vi "LC Global.vi"(7 "Mode":T3, 8 "error in (no error)":errorcluster caption="Error In", 9 "Write":T1) -> (0 "error out":errorcluster caption="Error Out", 2 "Read":T1[](array[typedef]), 3 "VI Info":T2)   [LabVIEW 2020]
uses:
  LC Mode.ctl
  LC Single Control Information.ctl
  LC Control Information.ctl
  <vilib>/Utility/xml.llb/Read From XML File(string).vi
  <vilib>/Utility/xml.llb/Write to XML File(string).vi
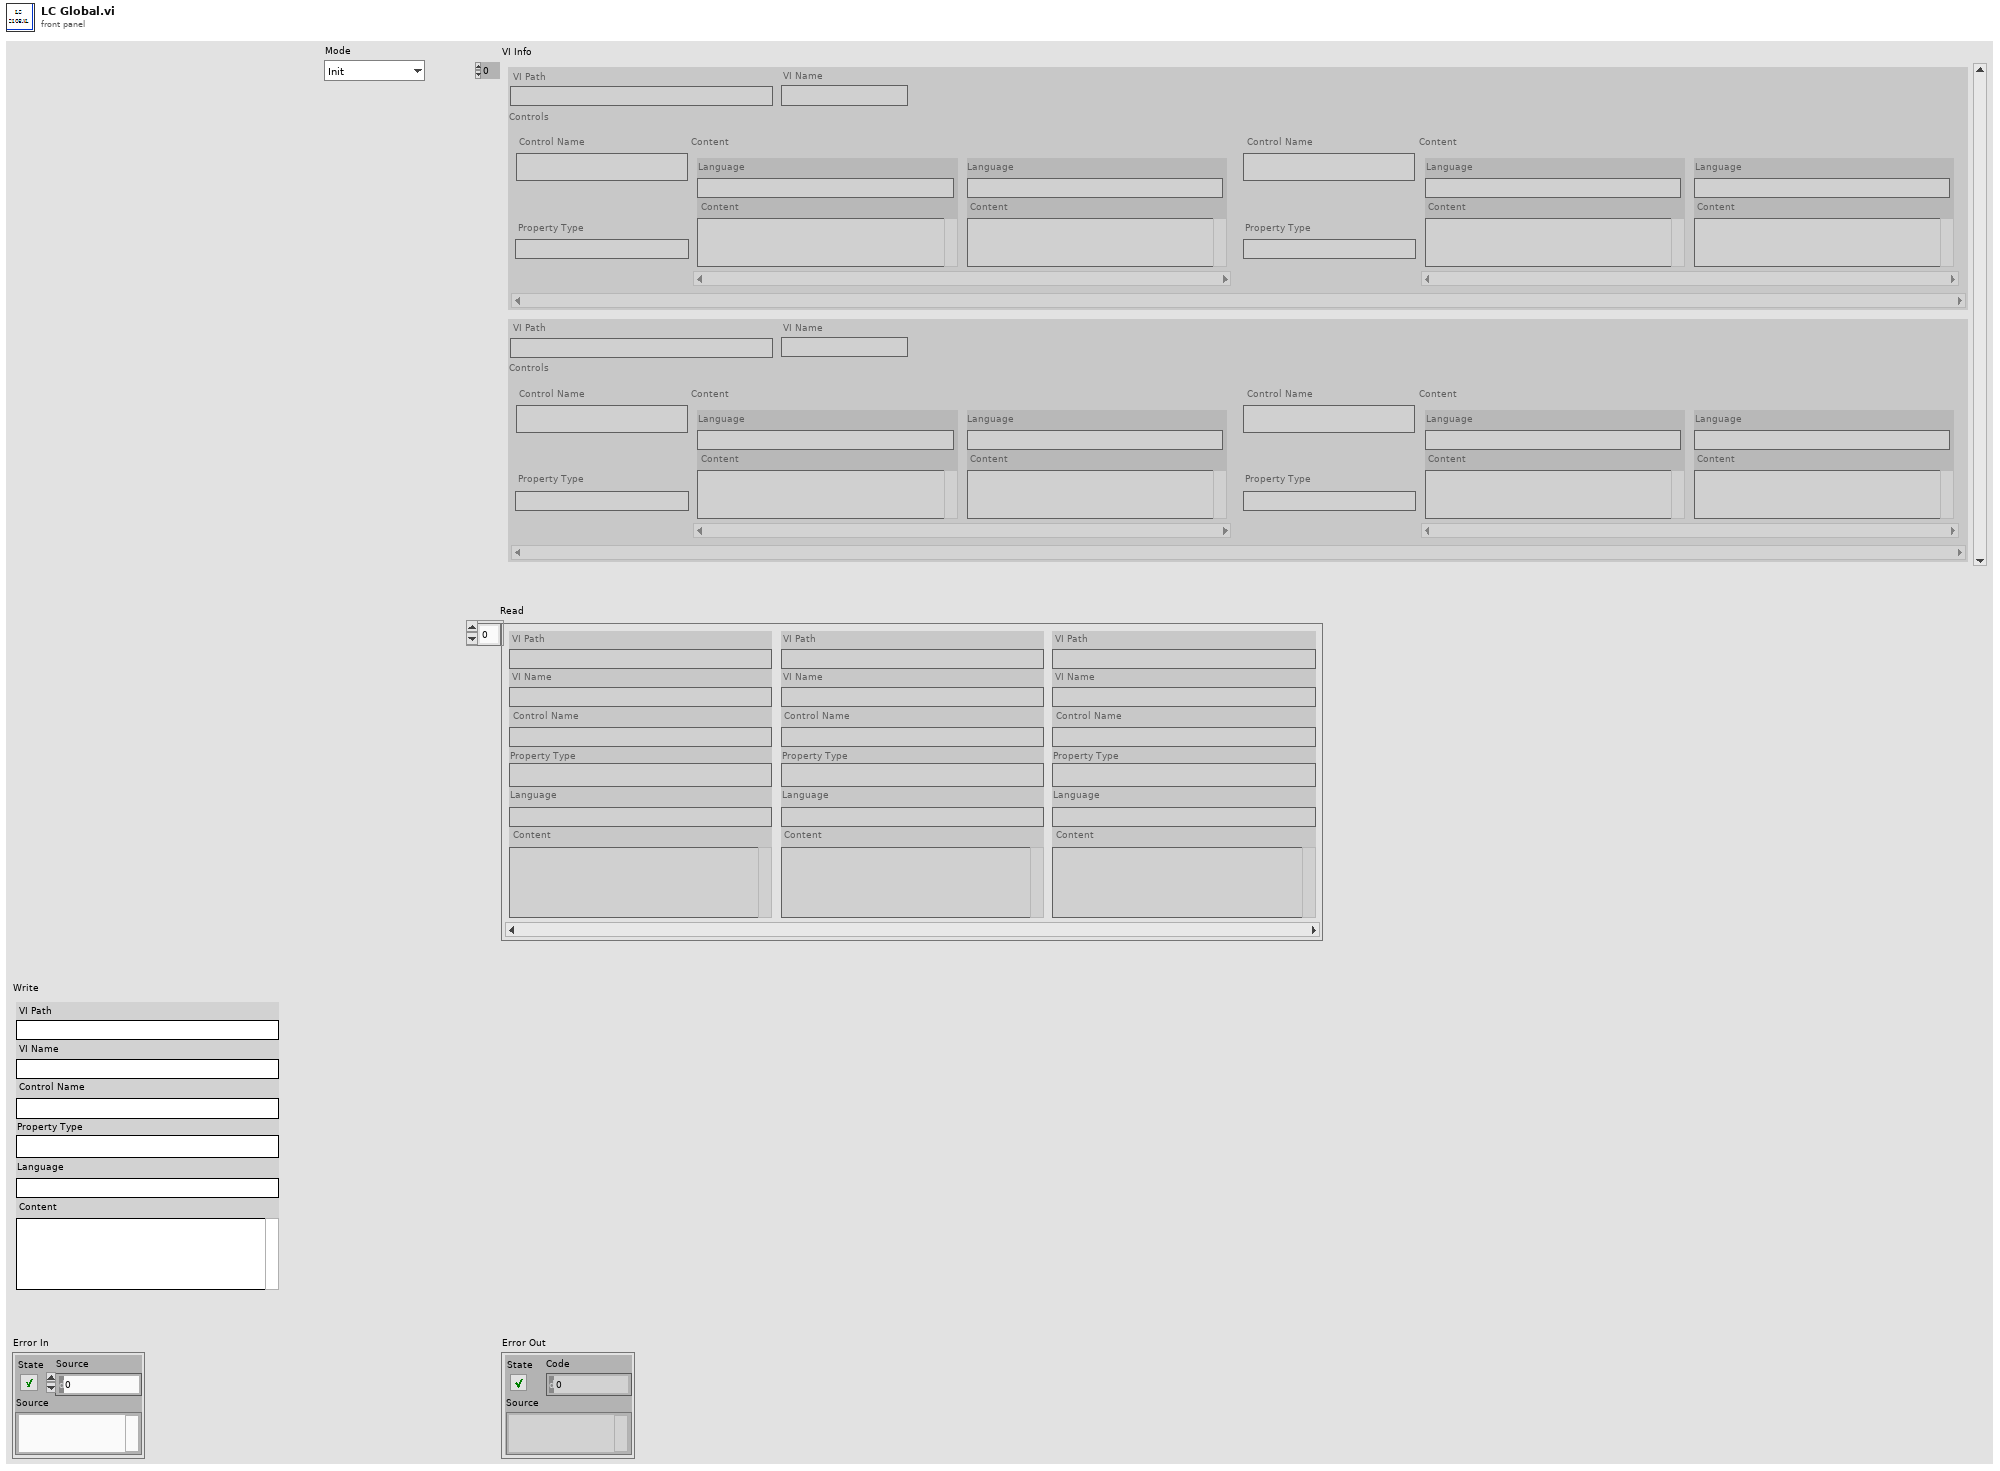
[diagram p1: front panel]
types:
  T1 = typedef "LC Single Control Information.ctl" = cluster{"VI Path":string, "VI Name":string, "Control Name":string, "Property Type":string, "Language":string, "Content":string}
  T2 = typedef "LC Control Information.ctl" = cluster{"Controls":cluster{"Control Name":string, "Property Type":string, "Content":cluster{"Language":string, "Content":string}[]}[], "VI Path":string, "VI Name":string}[]
  T3 = typedef "LC Mode.ctl" = enum16{"Init", "NONE", "Read", "Write", "Delete", "Clear", "Save"}
  T4 = cluster{"Control Name":string, "Property Type":string, "Content":cluster{"Language":string, "Content":string}[]}[]
  T5 = cluster{"Controls":cluster{"Control Name":string, "Property Type":string, "Content":cluster{"Language":string, "Content":string}[]}[], "VI Path":string, "VI Name":string}
  T6 = cluster{"Control Name":string, "Property Type":string, "Content":cluster{"Language":string, "Content":string}[]}
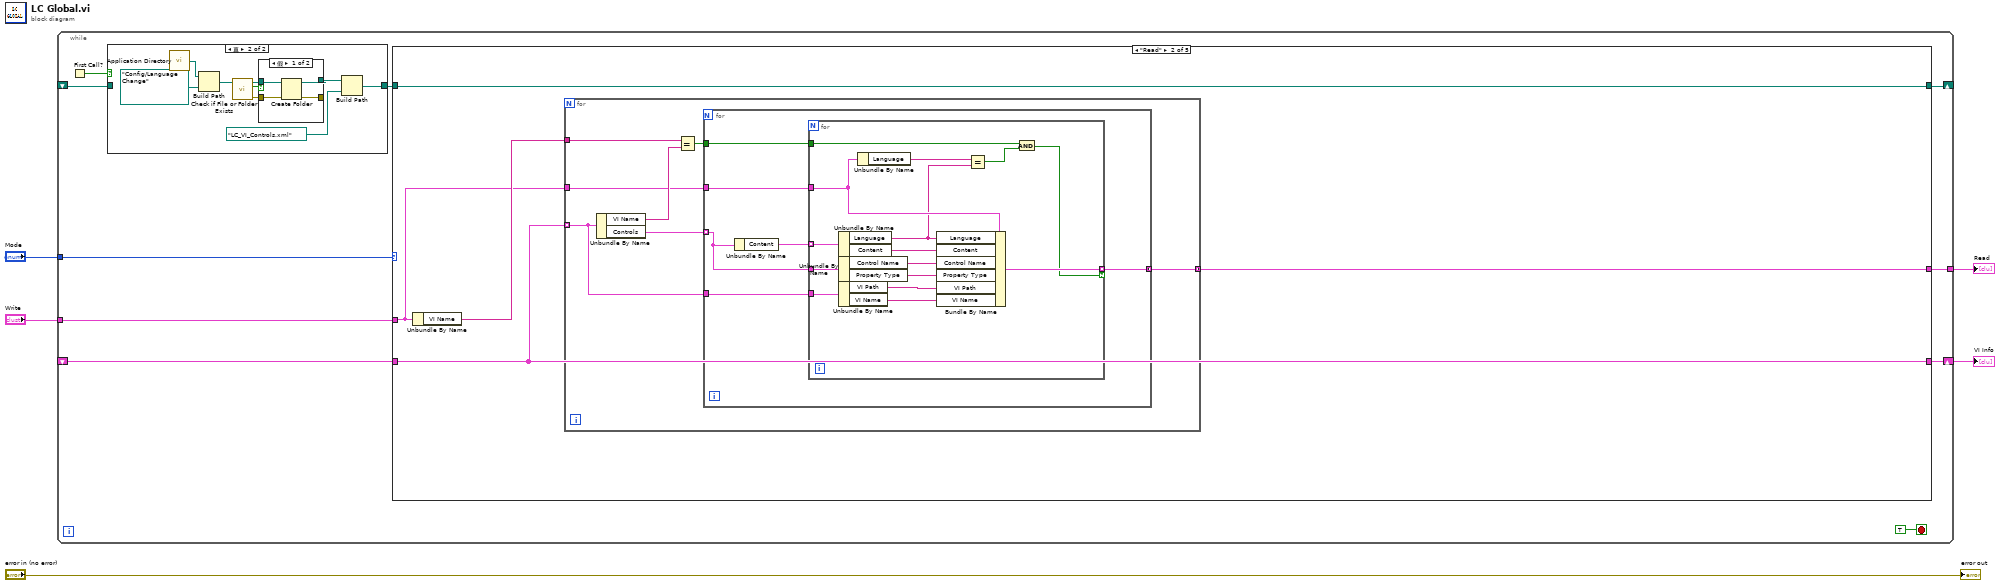
[diagram p0: block diagram]
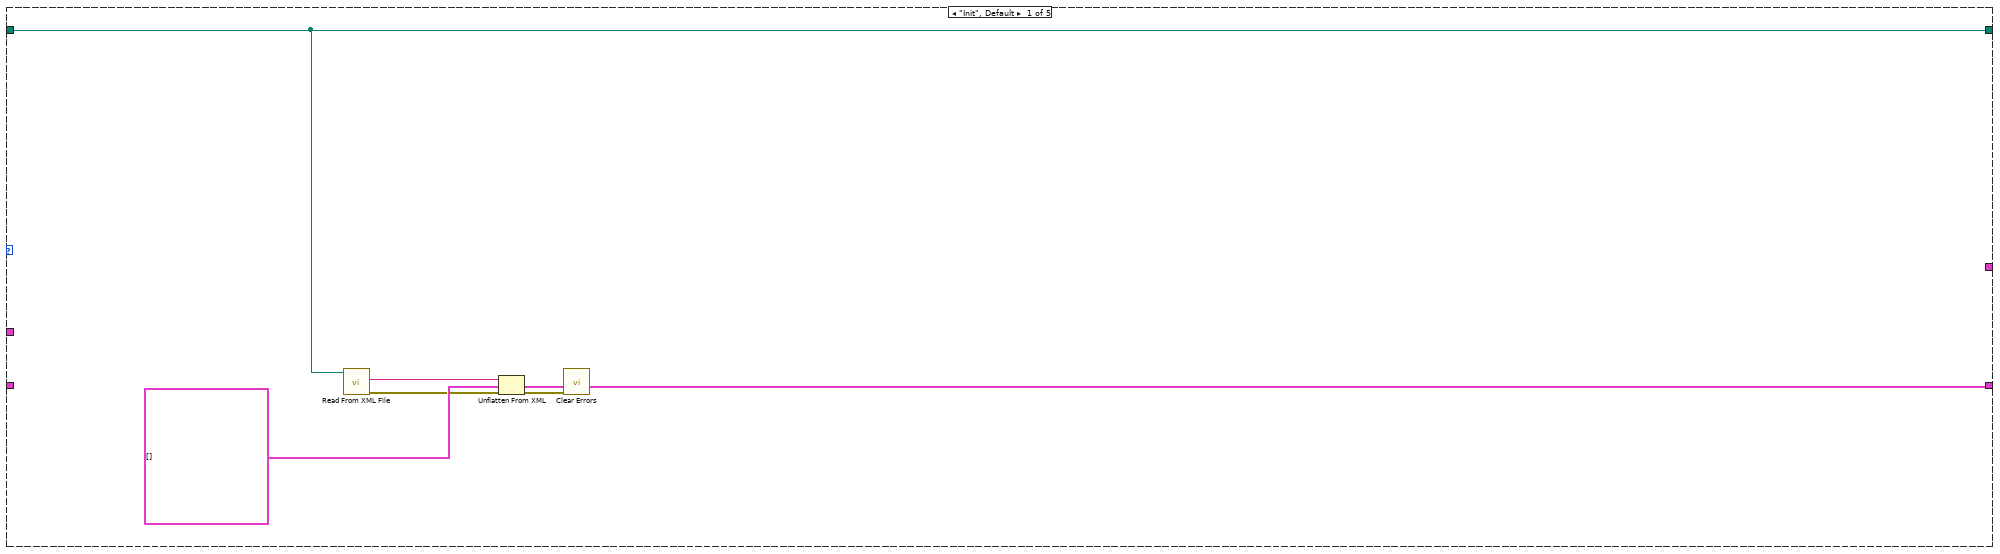
[diagram p4: hidden frame]
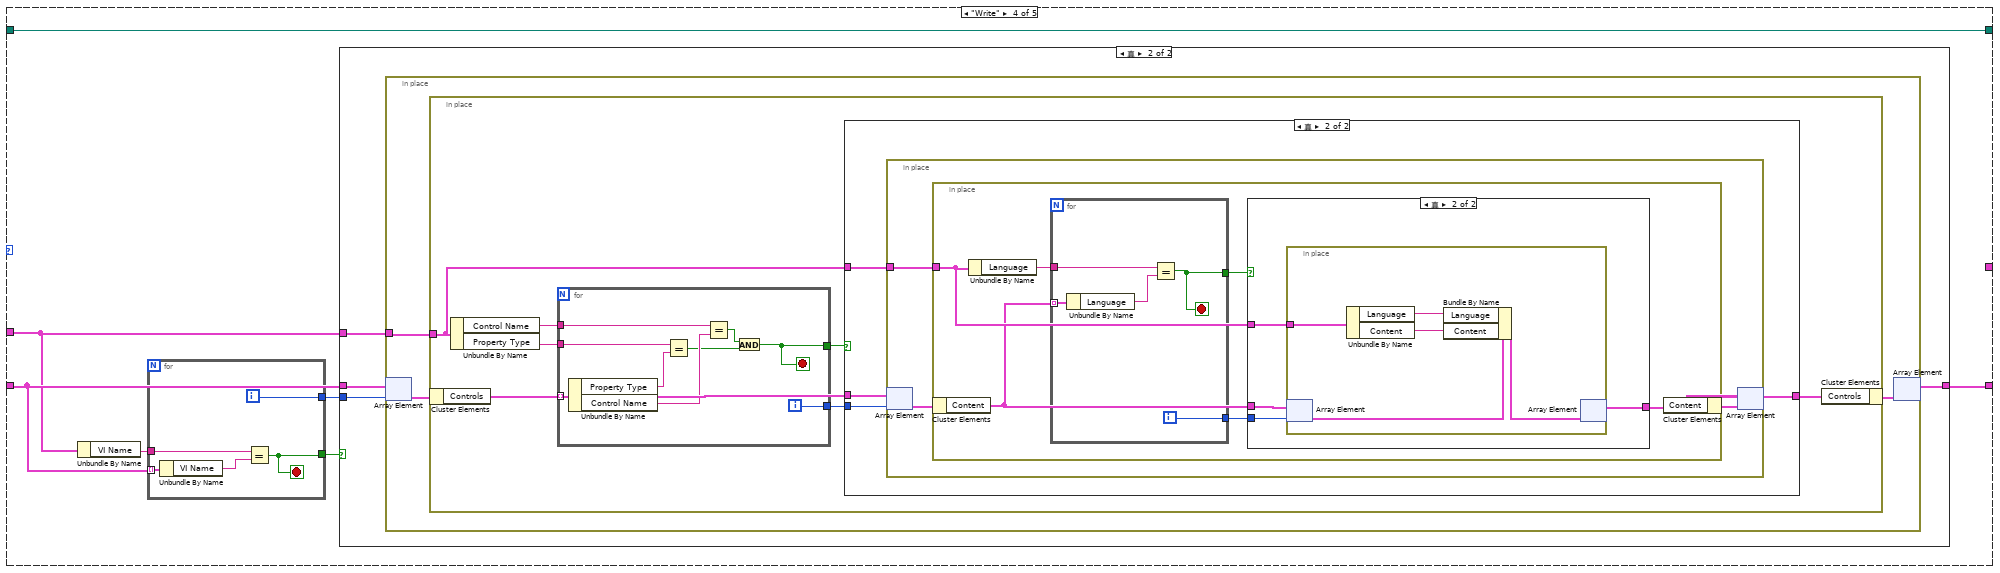
[diagram p6: hidden frame]
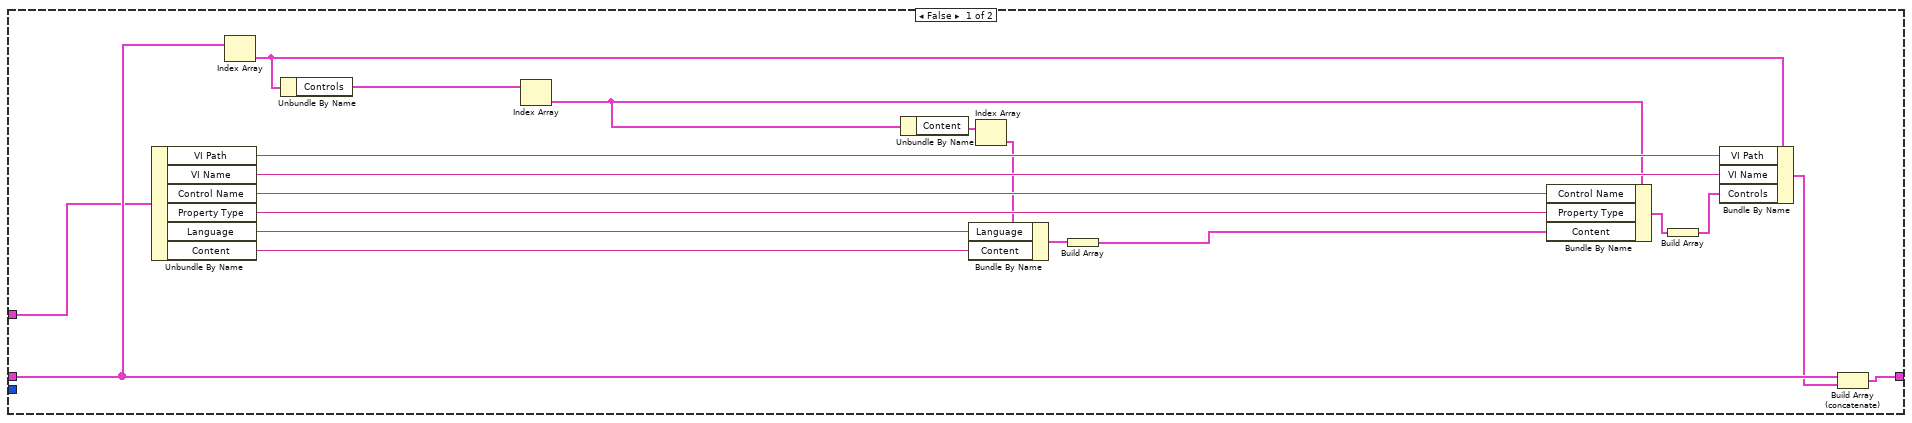
[diagram p7: hidden frame]
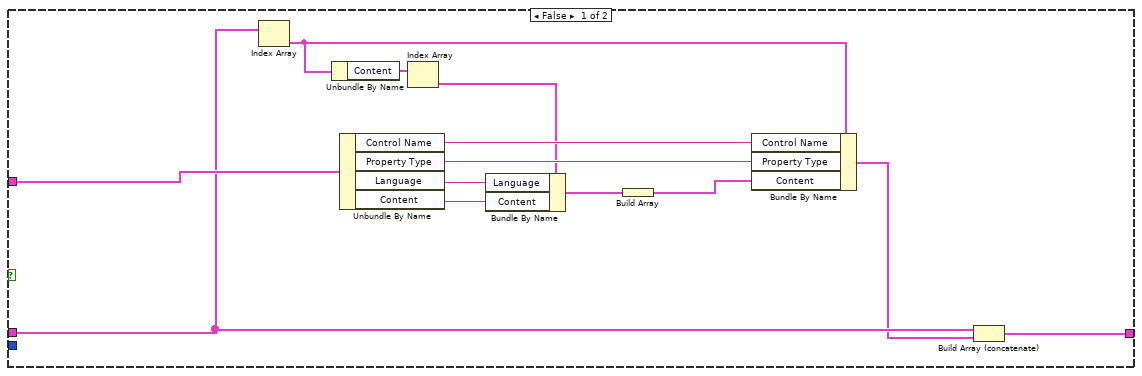
[diagram p8: hidden frame]
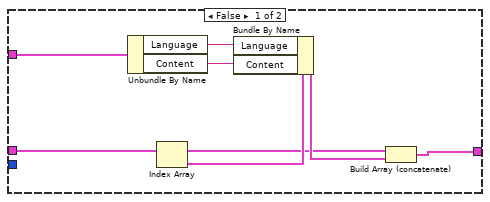
[diagram p9: hidden frame]
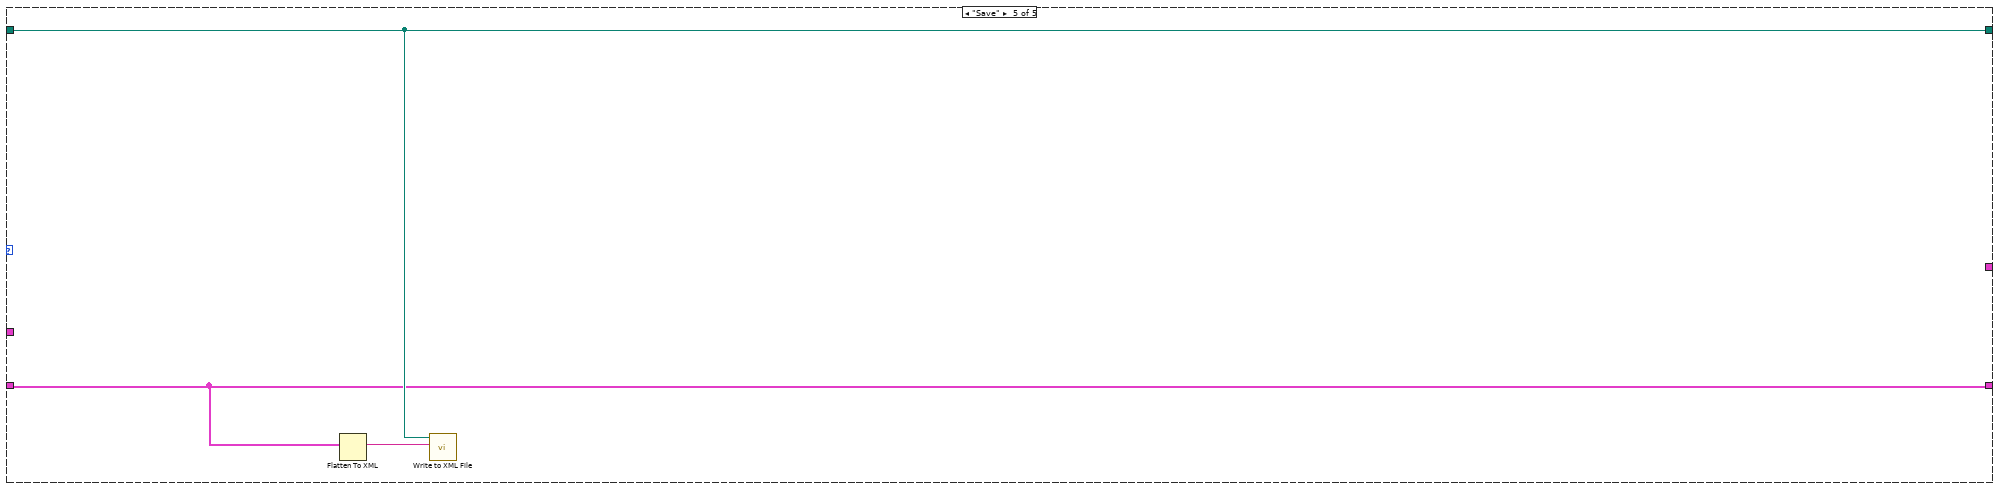
[diagram p10: hidden frame]
diagram:
  n1 = while {
    tunnel: "Mode" -> [w15]
    shift-right: [w13] -> _
    shift-left: _ -> [w8]
    shift-right: [w12] -> w2
    shift-left: _ -> [w11]
    tunnel: "Write" -> [w7]
    tunnel: [w6] -> w1
    stop <- TRUE stop-if-true
    n2 = First Call?() -> (First Call?: T/F=w10:bool)
    n3 = case shown="真" w10 {
      tunnel: [w16 w17] -> w9
      tunnel: w8 -> [w16 _]
      frame False {
      }
      frame True {
        n4 = call <vilib>:"Application Directory.vi"() -> ("Application Directory"=w25:path)
        n5 = Build Path(base path=w25, name or relative path=path "Config/Language Change" ("名称或相对路径")) -> (appended path=w23:path)
        n6 = call <vilib>:"Check if File or Folder Exists.vi"("path"=w23) -> ("error out"=w20:errorcluster, "file or folder exists?"=w22:bool, "dup path"=w21:path)  [unwired: 8 in]
        n7 = case shown="假" w22 {
          tunnel: w21 -> [w29 w31]
          tunnel: w20 -> [w28 w30]
          tunnel: [w27 w31] -> w19
          tunnel: [w26 w30] -> _
          frame False {
            n8 = Create Folder(path (use dialog)=w29, error in=w28) -> (created path=w27:path, error out=w26:errorcluster)  [unwired: 1 in, 1 out]
          }
          frame True {
          }
        }
        n9 = Build Path(base path=w19, name or relative path=path "LC_VI_Controls.xml" ("名称或相对路径")) -> (appended path=w17:path)
      }
    }
    n10 = case shown="\"Read\"" w15 {
      tunnel: [w37 w42 w72 w79 w175] -> w13
      tunnel: w9 -> [w37 w42 w72 w79 w175]
      tunnel: [w35 w40 w71 w73 w174] -> w12
      tunnel: w11 -> [_ w40 w71 w76 w174]
      tunnel: w7 -> [_ w39 _ w74 _]
      tunnel: [_ w38 _ _ _] -> w6
      frame "Init", Default {
        n11 = call-poly <vilib>:"Read From XML File.vi"("XML File Path"=w37) -> ("error out"=w33:errorcluster, "XML Elements"=w36:string)  [unwired: 8 in, 1 out]
        n12 = Unflatten From XML(xml string=w36, type=T2 [] ("VI Info"), error in (no error)=w33) -> (value=w35:T2, error out=w32:errorcluster)
        n13 = call <vilib>:"Clear Errors.vi"("error in (no error)"=w32) -> ()  [unwired: 5 in, 2 out]
      }
      frame "Read" {
        n14 = Unbundle By Name(w39) -> ("VI Name"=w41:string)
        n15 = for {
          tunnel: w41 -> [w48]
          tunnel: w40 -> [w44] mode=indexing
          tunnel: w39 -> [w45]
          tunnel: [w43] -> w38 mode=concatenating
          n16 = Unbundle By Name(w44) -> ("VI Name"=w49:string, "Controls"=w47:T4)
          n17 = Equal?(x=w48, y=w49) -> (x = y?=w46:bool)
          n18 = for {
            tunnel: w47 -> [w53] mode=indexing
            tunnel: w46 -> [w51]
            tunnel: w45 -> [w54]
            tunnel: w44 -> [w52]
            tunnel: [w50] -> w43 mode=concatenating
            n19 = Unbundle By Name(w53) -> ("Content"=w55:cluster{"Language":string, "Content":string}[])
            n20 = for {
              tunnel: w55 -> [w70] mode=indexing
              tunnel: w54 -> [w62]
              tunnel: w53 -> [w68]
              tunnel: w52 -> [w65]
              tunnel: w51 -> [w58]
              tunnel: [w57] -> w50 mode=indexing if=w56
              n21 = Unbundle By Name(w70) -> ("Language"=w60:string, "Content"=w69:string)
              n22 = Unbundle By Name(w68) -> ("Control Name"=w67:string, "Property Type"=w66:string)
              n23 = Unbundle By Name(w65) -> ("VI Path"=w64:string, "VI Name"=w63:string)
              n24 = Unbundle By Name(w62) -> ("Language"=w61:string)
              n25 = Bundle By Name(cluster=w62, "Language"=w60, "Content"=w69, "Control Name"=w67, "Property Type"=w66, "VI Path"=w64, "VI Name"=w63) -> (w57:T1)
              n26 = Equal?(x=w61, y=w60) -> (x = y?=w59:bool)
              n27 = And(x=w58, y=w59) -> (x .and. y?=w56:bool)
            }
          }
        }
      }
      frame "NONE" {
      }
      frame "Write" {
        n28 = Unbundle By Name(w74) -> ("VI Name"=w78:string)
        n29 = for {
          tunnel: w76 -> [w173] mode=indexing
          tunnel: w78 -> [w172]
          tunnel: [w170] -> w77
          tunnel: [w169] -> w75
          i -> [w169]
          stop <- w170 stop-if-true
          n30 = Unbundle By Name(w173) -> ("VI Name"=w171:string)
          n31 = Equal?(x=w172, y=w171) -> (x = y?=w170:bool)
        }
        n32 = case shown="真" w77 {
          tunnel: w76 -> [w98 w102]
          tunnel: w75 -> [_ w101]
          tunnel: w74 -> [w97 w100]
          tunnel: [w80 w99] -> w73
          frame False {
            n33 = Unbundle By Name(w97) -> ("VI Path"=w96:string, "VI Name"=w95:string, "Control Name"=w92:string, "Property Type"=w91:string, "Language"=w87:string, "Content"=w86:string)
            n34 = Index Array(array=w98) -> (element=w94:T5)  [unwired: 1 in]
            n35 = Unbundle By Name(w94) -> ("Controls"=w93:T4)
            n36 = Index Array(array=w93) -> (element=w90:T6)  [unwired: 1 in]
            n37 = Unbundle By Name(w90) -> ("Content"=w89:cluster{"Language":string, "Content":string}[])
            n38 = Index Array(array=w89) -> (element=w88:cluster{"Language":string, "Content":string})  [unwired: 1 in]
            n39 = Bundle By Name(cluster=w88, "Language"=w87, "Content"=w86) -> (w85:cluster{"Language":string, "Content":string})
            n40 = Build Array(w85) -> (w84:cluster{"Language":string, "Content":string}[])
            n41 = Bundle By Name(cluster=w90, "Control Name"=w92, "Property Type"=w91, "Content"=w84) -> (w83:T6)
            n42 = Build Array(w83) -> (w82:T4)
            n43 = Bundle By Name(cluster=w94, "VI Path"=w96, "VI Name"=w95, "Controls"=w82) -> (w81:T5)
            n44 = Build Array (concatenate)(w98, w81) -> (w80:T2)
          }
          frame True {
            n45 = in-place {
              in-place-border: w100 -> [w105]
              n46 = in-place-array #1(w102, w101) -> (w104:T5)
              n47 = in-place {
                in-place-border: w105 -> [w109]
                n48 = in-place-cluster #2(w104) -> ("Controls"=w107:T4)
                n49 = Unbundle By Name(w109) -> ("Control Name"=w112:string, "Property Type"=w108:string)
                n50 = for {
                  tunnel: w107 -> [w168] mode=indexing
                  tunnel: w112 -> [w167]
                  tunnel: [w165] -> w110
                  tunnel: [w160] -> w111
                  tunnel: w108 -> [w164]
                  i -> [w165]
                  stop <- w160 stop-if-true
                  n51 = Unbundle By Name(w168) -> ("Property Type"=w163:string, "Control Name"=w166:string)
                  n52 = Equal?(x=w164, y=w163) -> (x = y?=w161:bool)
                  n53 = Equal?(x=w167, y=w166) -> (x = y?=w162:bool)
                  n54 = And(x=w162, y=w161) -> (x .and. y?=w160:bool)
                }
                n55 = case shown="真" w111 {
                  tunnel: w110 -> [_ w127]
                  tunnel: w107 -> [w115 w128]
                  tunnel: w109 -> [w125 w129]
                  tunnel: [w113 w126] -> w106
                  frame False {
                    n56 = Index Array(array=w115) -> (element=w122:T6)  [unwired: 1 in]
                    n57 = Unbundle By Name(w122) -> ("Content"=w121:cluster{"Language":string, "Content":string}[])
                    n58 = Unbundle By Name(w125) -> ("Control Name"=w124:string, "Property Type"=w123:string, "Language"=w119:string, "Content"=w118:string)
                    n59 = Index Array(array=w121) -> (element=w120:cluster{"Language":string, "Content":string})  [unwired: 1 in]
                    n60 = Bundle By Name(cluster=w120, "Language"=w119, "Content"=w118) -> (w117:cluster{"Language":string, "Content":string})
                    n61 = Build Array(w117) -> (w116:cluster{"Language":string, "Content":string}[])
                    n62 = Bundle By Name(cluster=w122, "Control Name"=w124, "Property Type"=w123, "Content"=w116) -> (w114:T6)
                    n63 = Build Array (concatenate)(w115, w114) -> (w113:T4)
                  }
                  frame True {
                    n64 = in-place {
                      in-place-border: w129 -> [w132]
                      n65 = in-place-array #3(w128, w127) -> (w131:T6)
                      n66 = in-place {
                        in-place-border: w132 -> [w138]
                        n67 = in-place-cluster #4(w131) -> ("Content"=w134:cluster{"Language":string, "Content":string}[])
                        n68 = Unbundle By Name(w138) -> ("Language"=w137:string)
                        n69 = for {
                          tunnel: w134 -> [w143] mode=indexing
                          tunnel: w137 -> [w142]
                          tunnel: [w140] -> w135
                          tunnel: [w139] -> w136
                          i -> [w140]
                          stop <- w139 stop-if-true
                          n70 = Unbundle By Name(w143) -> ("Language"=w141:string)
                          n71 = Equal?(x=w142, y=w141) -> (x = y?=w139:bool)
                        }
                        n72 = case shown="真" w136 {
                          tunnel: w135 -> [_ w153]
                          tunnel: w134 -> [w144 w154]
                          tunnel: w138 -> [w150 w152]
                          tunnel: [w145 w151] -> w133
                          frame False {
                            n73 = Unbundle By Name(w150) -> ("Language"=w148:string, "Content"=w147:string)
                            n74 = Index Array(array=w144) -> (element=w149:cluster{"Language":string, "Content":string})  [unwired: 1 in]
                            n75 = Bundle By Name(cluster=w149, "Language"=w148, "Content"=w147) -> (w146:cluster{"Language":string, "Content":string})
                            n76 = Build Array (concatenate)(w144, w146) -> (w145:cluster{"Language":string, "Content":string}[])
                          }
                          frame True {
                            n77 = in-place {
                              in-place-border: w152 -> [w158]
                              n78 = in-place-array #5(w154, w153) -> (w159:cluster{"Language":string, "Content":string})
                              n79 = Unbundle By Name(w158) -> ("Language"=w157:string, "Content"=w156:string)
                              n80 = Bundle By Name(cluster=w159, "Language"=w157, "Content"=w156) -> (w155:cluster{"Language":string, "Content":string})
                              n81 = in-place-array #5(w155) -> (w151:cluster{"Language":string, "Content":string}[])  [unwired: 1 out]
                            }
                          }
                        }
                        n82 = in-place-cluster #4("Content"=w133) -> (w130:T6)
                      }
                      n83 = in-place-array #3(w130) -> (w126:T4)  [unwired: 1 out]
                    }
                  }
                }
                n84 = in-place-cluster #2("Controls"=w106) -> (w103:T5)
              }
              n85 = in-place-array #1(w103) -> (w99:T2)  [unwired: 1 out]
            }
          }
        }
      }
      frame "Save" {
        n86 = Flatten To XML(6:w174) -> (2:w176:string)
        n87 = call-poly <vilib>:"Write to XML File.vi"("XML Input"=w176, "XML File Path"=w175) -> ()  [unwired: 7 in, 3 out]
      }
    }
  }
  "VI Info" <- w2
  "Read" <- w1
  "error out" <- "error in (no error)"
